vi "Update_FFID_Bkgnd_info.vi"(1 "First Bknd since calib":bool, 2 "c^2 (ppm^2)":dbl[](array[numeric]), 3 "Specific Bkgnd Meas?":bool, 4 "C (ppm)":dbl[](array[numeric])) -> ()   [LabVIEW 2021]
uses:
  Globals/Meas_global.vi
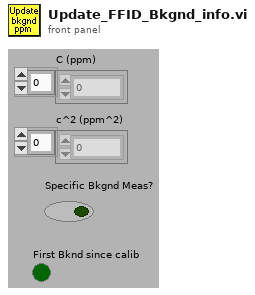
[diagram p1: front panel]
types:
  T1 = typedef "Analysis_info_cluster.ctl" = cluster{"Colour":u32, "Inst type":T2, "Inst name":string, "Symbol":string, "Code name":string, "Extra Info":string, "Inst Array":T3, "Extra Titles":string[], "Extra Values":string[], "U":dbl, "u^2":dbl, "u^3":dbl, "u^4":dbl, "Skew_u":dbl, "Kurt_u":dbl, "Sd Error in Mean":dbl, "% u'/U":dbl, "X":dbl, "Y":dbl, "Z":dbl, "Timescale integral Estimate":dbl, "Sd Error in Variance":dbl, "Calib File":path, "Calib Constants":dbl[], "Output Position":bool, "Stats":enum16{"None", "Basic", "Full"}, "Av Sampling Rate":dbl, "Av No of Samples":dbl, "Total Meas Time (s)":dbl, "ADAM Ch Name":string, "Max value":dbl, "Min value":dbl, "Req Sample Rate Hz":dbl, "Sync Delay Time (s)":dbl, "Ch No":i16, "Device":string, "Use Latest Calib":bool, "Port":string, "Metadata Ch Names":string[], "Metadata Ch Values":string[], "Label":string}
  T2 = typedef "Inst_type.ctl" = enum16{"Raw voltage", "Raw with zero offsetting", "Propeller anemometer", "Pressure Transducer", "Pitot-static tube", "Hot wire", "Cross wire 1", "Cross wire 2", "Generic Linear", "Generic Polynomial", "Generic BackPoly", "Fast FID", "Thermocouple", "Cold wire", "Pulsed Wire", "LDA Vel", "LDA Tran time", "LDA Arr time", "Microphone"}
  T3 = typedef "Instrument_Array.ctl" = enum16{"PWA", "LDA", "Analogue"}
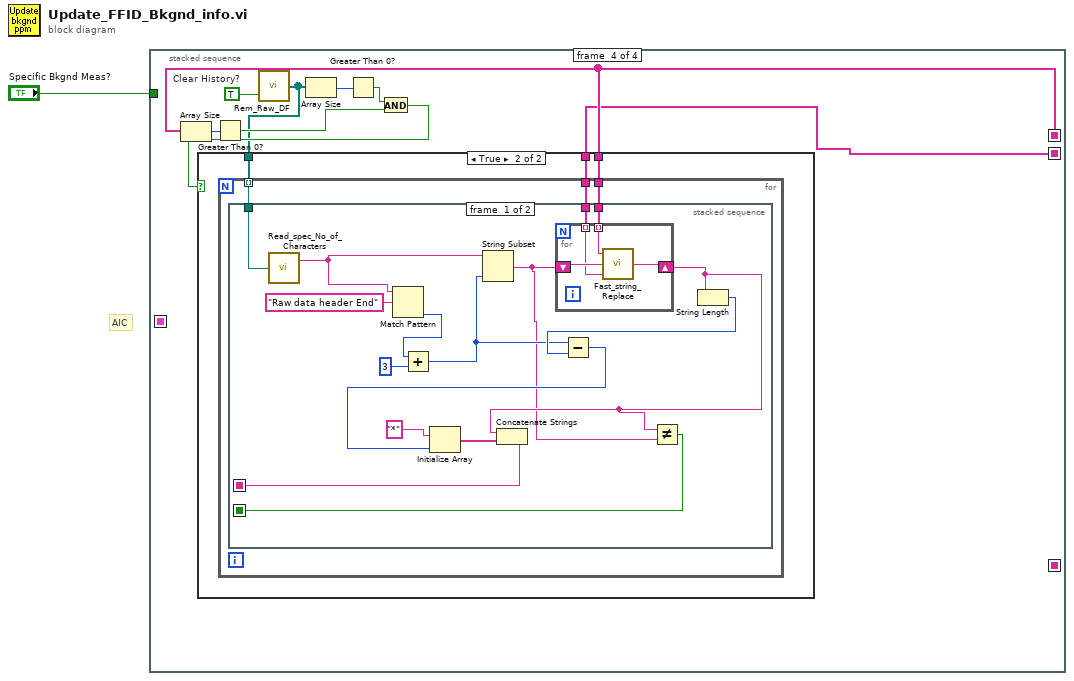
[diagram p0: block diagram]
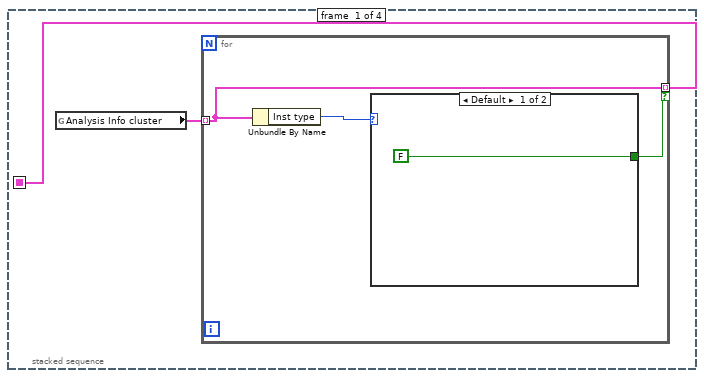
[diagram p2: hidden frame]
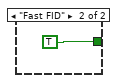
[diagram p3: hidden frame]
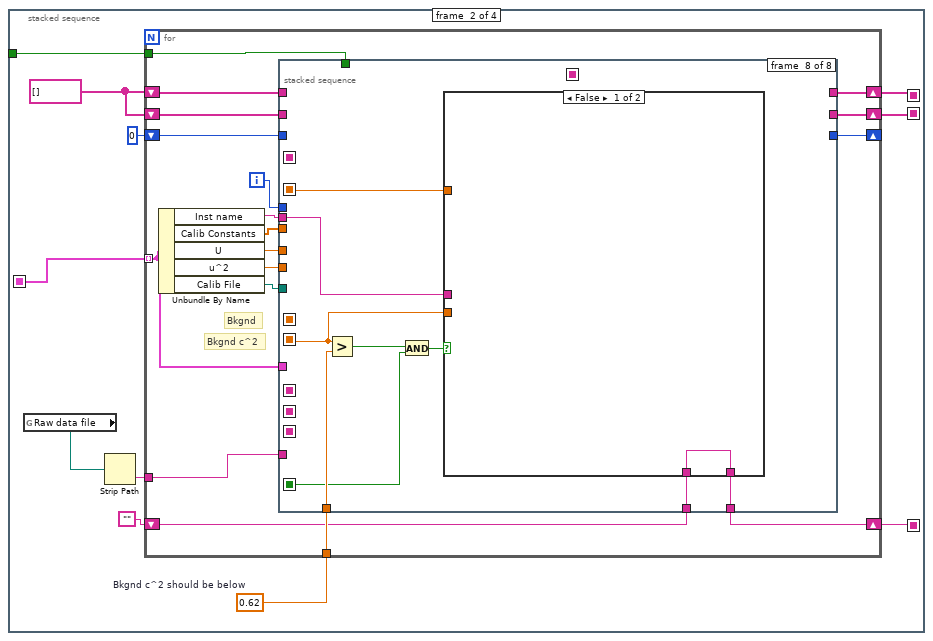
[diagram p4: hidden frame]
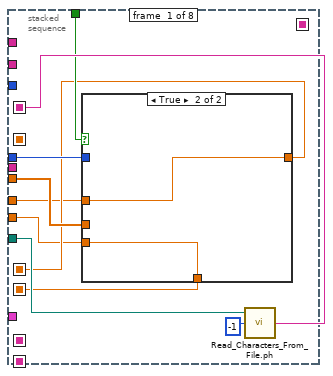
[diagram p5: hidden frame]
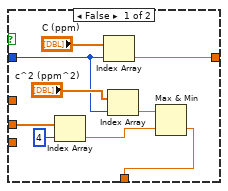
[diagram p6: hidden frame]
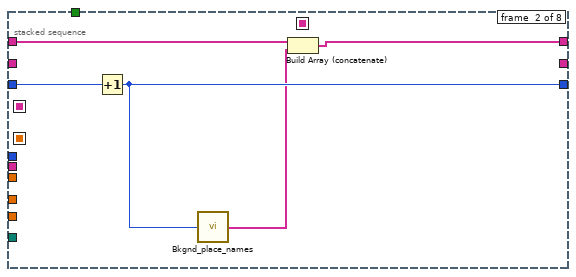
[diagram p7: hidden frame]
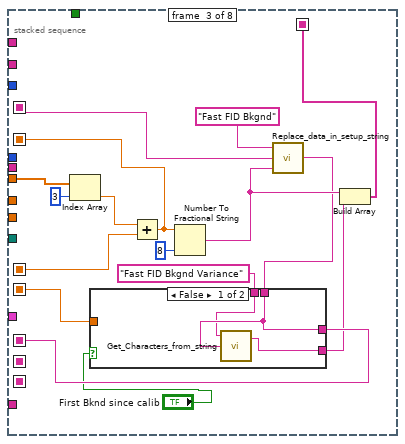
[diagram p8: hidden frame]
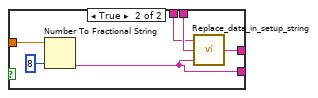
[diagram p9: hidden frame]
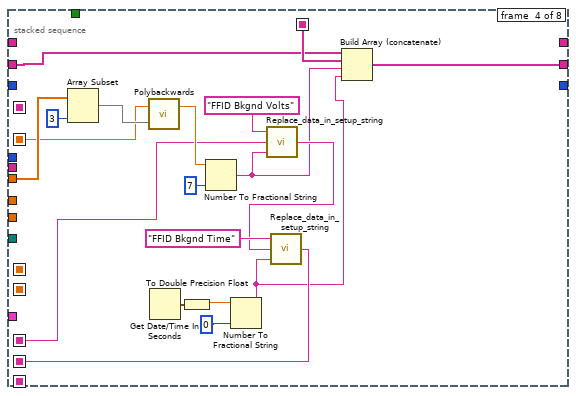
[diagram p10: hidden frame]
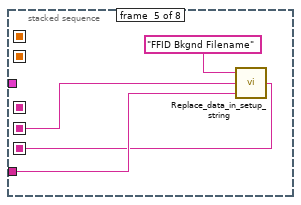
[diagram p11: hidden frame]
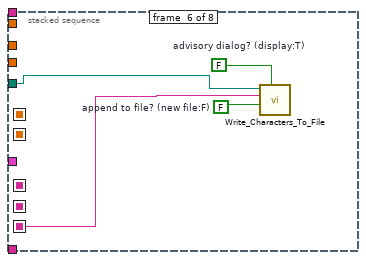
[diagram p12: hidden frame]
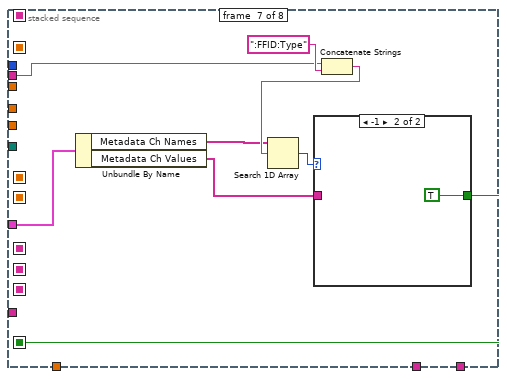
[diagram p13: hidden frame]
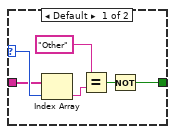
[diagram p14: hidden frame]
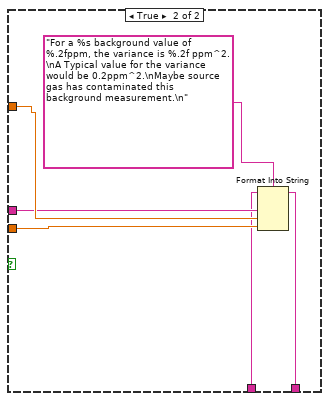
[diagram p15: hidden frame]
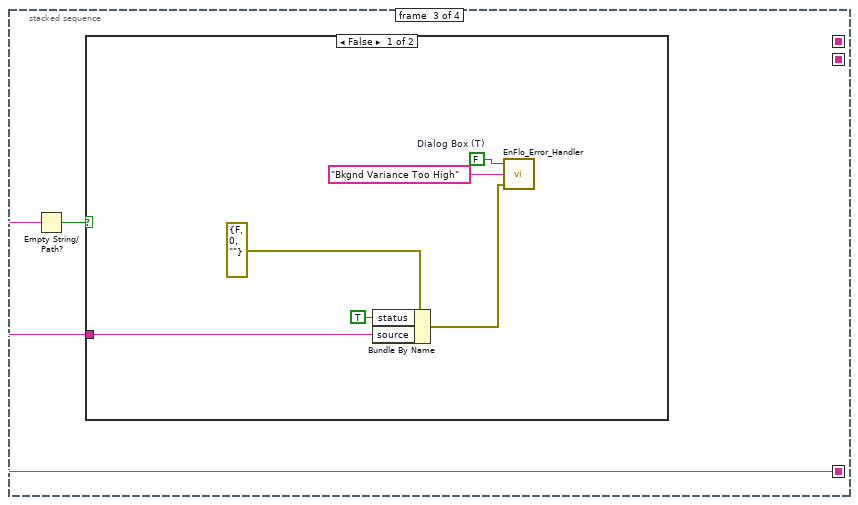
[diagram p16: hidden frame]
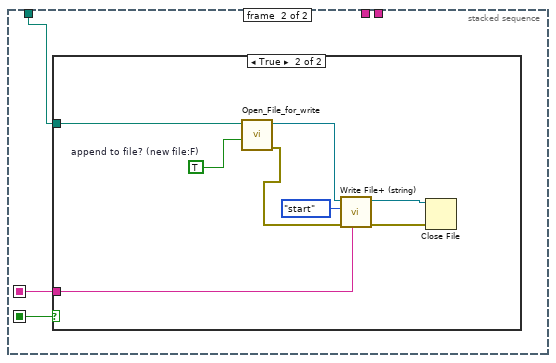
[diagram p19: hidden frame]
diagram:
  # "AIC"
  n1 = stacked-sequence {
    seq-local: [_ w15 _ _] -> [_ _ _ w157]
    seq-local: [_ w14 _ _] -> [_ _ _ w156]
    seq-local: [w2 _ _ _] -> [_ w12 _ _]
    seq-local: [_ w9 _ _] -> [_ _ w147 _]
    tunnel: "Specific Bkgnd Meas?" -> [_ w11 _ _]
    frame #0 {
      n2 = global read "Meas_global.vi" "Analysis Info cluster"() -> (w3:T1[])
      n3 = for {
        tunnel: w3 -> [w6] mode=indexing
        tunnel: [w6] -> w2 mode=indexing if=w4
        n4 = Unbundle By Name(w6) -> ("Inst type"=w5:T2)
        n5 = case shown="Default" w5 {
          tunnel: [FALSE TRUE] -> w4
          frame Default {
          }
          frame "Fast FID" {
          }
        }
      }
    }
    frame #1 {
      w13 = 0.62  # Bkgnd c^2 should be below
      w16 = string[] []
      n6 = global read "Meas_global.vi" "Raw data file"() -> (w19:path)
      n7 = Strip Path(path=w19) -> (name=w18:string)  [unwired: 1 out]
      n8 = for {
        tunnel: w18 -> [w37]
        shift-right: [w35] -> _
        shift-left: 0 -> [w36]
        shift-right: [w31] -> w14
        shift-left: w16 -> [w32]
        shift-right: [w33] -> w15
        shift-left: w16 -> [w34]
        tunnel: w13 -> [w30]
        tunnel: w12 -> [w22] mode=indexing
        tunnel: w11 -> [w29]
        shift-right: [w20] -> w9
        shift-left: "" -> [w21]
        i -> [w28]
        # "Bkgnd c^2"
        # "Bkgnd"
        n9 = Unbundle By Name(w22) -> ("Inst name"=w23:string, "Calib Constants"=w27:dbl[], "U"=w26:dbl, "u^2"=w24:dbl, "Calib File"=w25:path)
        n10 = stacked-sequence {
          seq-local: [w46 _ _ _ _ _ _ _] -> [_ _ w74 _ _ _ _ _]
          seq-local: [_ _ w73 _ _ _ _ _] -> [_ _ _ w96 _ _ _ _]
          seq-local: [_ _ w72 _ _ _ _ _] -> [_ _ _ w104 _ _ _ w139]
          seq-local: [_ _ _ w94 _ _ _ _] -> [_ _ _ _ w108 _ _ _]
          seq-local: [_ _ _ _ w109 _ _ _] -> [_ _ _ _ _ w113 _ _]
          seq-local: [_ _ w68 _ _ _ _ _] -> [_ _ _ w93 _ _ _ _]
          seq-local: [w43 _ _ _ _ _ _ _] -> [_ _ w67 _ _ _ _ w138]
          seq-local: [w40 _ _ _ _ _ _ _] -> [_ _ w66 _ _ _ _ _]
          seq-local: [_ _ _ _ _ _ w116 _] -> [_ _ _ _ _ _ _ w134]
          tunnel: w27 -> [w42 _ w79 w107 _ _ _ _]
          tunnel: w25 -> [w45 _ _ _ _ w112 _ _]
          tunnel: w37 -> [_ _ _ _ w110 _ _ _]
          tunnel: w36 -> [_ w63 _ _ _ _ _ _]
          tunnel: [_ w62 _ _ _ _ _ _] -> w35
          tunnel: w34 -> [_ w60 _ _ _ _ _ _]
          tunnel: [_ w59 _ _ _ _ _ _] -> w33
          tunnel: w32 -> [_ _ _ w90 _ _ _ _]
          tunnel: [_ _ _ w89 _ _ _ _] -> w31
          tunnel: w30 -> [_ _ _ _ _ _ _ w137]
          tunnel: w29 -> [w44 _ _ _ _ _ _ _]
          tunnel: w28 -> [w41 _ _ _ _ _ _ _]
          tunnel: w26 -> [w39 _ _ _ _ _ _ _]
          tunnel: w24 -> [w38 _ _ _ _ _ _ _]
          tunnel: w23 -> [_ _ _ _ _ _ w117 w136]
          tunnel: w22 -> [_ _ _ _ _ _ w120 _]
          tunnel: w21 -> [_ _ _ _ _ _ _ w132]
          tunnel: [_ _ _ _ _ _ _ w131] -> w20
          frame #0 {
            n11 = case shown="True" w44 {
              tunnel: [w48 w57] -> w43
              tunnel: w42 -> [w56 _]
              tunnel: w41 -> [w51 _]
              tunnel: [w53 w58] -> w40
              tunnel: w39 -> [_ w58]
              tunnel: w38 -> [_ w57]
              frame False {
                n12 = Index Array(array=w56, index=4) -> (element=w49:dbl)
                n13 = Index Array(array="C (ppm)", index=w51) -> (element=w53:dbl)
                n14 = Index Array(array="c^2 (ppm^2)", index=w51) -> (element=w50:dbl)
                n15 = Max & Min(x=w50, y=w49) -> (min(x,y)=w48:dbl)  [unwired: 1 out]
              }
              frame True {
              }
            }
            n16 = call "Read_Characters_From_File.ph.vi"("file path (dialog if empty)"=w45, "number of characters (all:-1)"=-1) -> ("character string"=w46:string)  [unwired: 7 out]
          }
          frame #1 {
            n17 = Increment(x=w63) -> (x+1=w62:i32)
            n18 = call "Bkgnd_place_names.vi"("Numeric"=w62) -> ("Array"=w61:string[])
            n19 = Build Array (concatenate)(w60, w61) -> (w59:string[])
          }
          frame #2 {
            n20 = Index Array(array=w79, index=3 ("Index")) -> (element=w77:dbl)
            n21 = Add(x=w77, y=w66) -> (x+y=w72:dbl)
            n22 = Number To Fractional String(number=w72, precision (6)=i16 8) -> (F-format string=w71:string)  [unwired: 2 out]
            n23 = call "Replace_data_in_setup_string.vi"("New data string"=w71, "Input string"=w74, "Variable name"="Fast FID Bkgnd") -> ("Appended string"=w70:string)
            n24 = case shown="False" "First Bknd since calib" {
              tunnel: [w82 w88] -> w73
              tunnel: w70 -> [w82 w86]
              tunnel: [w80 w85] -> w69
              tunnel: w67 -> [_ w84]
              tunnel: "Fast FID Bkgnd Variance" -> [w81 w83]
              frame False {
                n25 = call "Get_Characters_from_string.vi"("Input string"=w82, "Variable name"=w81) -> ("Value"=w80:string)  [unwired: 1 in, 1 out]
              }
              frame True {
                n26 = Number To Fractional String(number=w84, precision (6)=i16 8) -> (F-format string=w85:string)  [unwired: 2 out]
                n27 = call "Replace_data_in_setup_string.vi"("New data string"=w85, "Input string"=w86, "Variable name"=w83) -> ("Appended string"=w88:string)
              }
            }
            n28 = Build Array(w71, w69) -> (w68:string[])
          }
          frame #3 {
            n29 = Array Subset(array=w107, length=3 ("index")) -> (w105:dbl[])  [unwired: 1 in]
            n30 = call "Polybackwards.vi"("Coefficients"=w105, "Y input"=w104) -> ("X output"=w103:dbl)  [unwired: 1 out]
            n31 = Get Date/Time In Seconds() -> (seconds since 1Jan1904=w100:timestamp)
            n32 = To Double Precision Float(number=w100) -> (double precision float=w98:dbl)
            n33 = Number To Fractional String(number=w103, precision (6)=i16 7) -> (F-format string=w92:string)  [unwired: 2 out]
            n34 = Number To Fractional String(number=w98, precision (6)=i16 0) -> (F-format string=w91:string)  [unwired: 2 out]
            n35 = call "Replace_data_in_setup_string.vi"("New data string"=w92, "Input string"=w96, "Variable name"="FFID Bkgnd Volts") -> ("Appended string"=w95:string)
            n36 = call "Replace_data_in_setup_string.vi"("New data string"=w91, "Input string"=w95, "Variable name"="FFID Bkgnd Time") -> ("Appended string"=w94:string)
            n37 = Build Array (concatenate)(w90, w93, w92, w91) -> (w89:string[])
          }
          frame #4 {
            n38 = call "Replace_data_in_setup_string.vi"("New data string"=w110, "Input string"=w108, "Variable name"="FFID Bkgnd Filename") -> ("Appended string"=w109:string)
          }
          frame #5 {
            w114 = FALSE  # advisory dialog? (display:T)
            w115 = FALSE  # append to file? (new file:F)
            n39 = call "Write_Characters_To_File.vi"("file path (dialog if empty)"=w112, "advisory dialog? (display:T)"=w114, "character string"=w113, "append to file? (new file:F)"=w115) -> ()  [unwired: 1 in, 4 out]
          }
          frame #6 {
            n40 = Unbundle By Name(w120) -> ("Metadata Ch Names"=w119:string[], "Metadata Ch Values"=w118:string[])
            n41 = Concatenate Strings(w117, ":FFID:Type" ("string")) -> (w122:string)
            n42 = Search 1D Array(1D array=w119, element=w122) -> (index of element=w121:i32)  [unwired: 1 in]
            n43 = case shown="-1" w121 {
              selector: w121 -> [w129 _]
              tunnel: [w124 TRUE] -> w116
              tunnel: w118 -> [w128 _]
              frame Default {
                n44 = Index Array(array=w128, index=w129) -> (element=w127:string)
                n45 = Equal?(x="Other", y=w127) -> (x = y?=w125:bool)
                n46 = Not(x=w125) -> (.not. x?=w124:bool)
              }
              frame -1 {
              }
            }
          }
          frame #7 {
            n47 = Greater?(x=w138, y=w137) -> (0:w135:bool)
            n48 = And(x=w135, y=w134) -> (x .and. y?=w133:bool)
            n49 = case shown="False" w133 {
              tunnel: w138 -> [_ w146]
              tunnel: w139 -> [_ w145]
              tunnel: w136 -> [_ w143]
              tunnel: w132 -> [w140 w142]
              tunnel: [w140 w141] -> w131
              frame False {
              }
              frame True {
                n50 = Format Into String(format string="For a %s background value of %.2fppm, the variance is %.2f ppm^2.\nA Typical value for the variance would be 0.2ppm^2.\nMaybe source gas has contaminated this background measurement.\n", initial string=w142, w143, w145, w146) -> (resulting string=w141:string)  [unwired: 1 in, 1 out]
              }
            }
          }
        }
      }
    }
    frame #2 {
      n51 = Empty String/Path?(string/path=w147) -> (empty?=w148:bool)
      n52 = case shown="False" w148 {
        tunnel: w147 -> [w150 _]
        frame False {
          w153 = FALSE  # Dialog Box (T)
          n53 = Bundle By Name(cluster=errorcluster {"status"=FALSE, "code"=0, "source"=""} ("error in (no error)"), "status"=TRUE, "source"=w150) -> (w149:errorcluster)
          n54 = call "EnFlo_Error_Handler.vi"("error in (no error)"=w149, "Error Type"="Bkgnd Variance Too High", "Dialog Box (F)"=w153) -> ()  [unwired: 3 out]
        }
        frame True {
        }
      }
    }
    frame #3 {
      w155 = TRUE  # Clear History?
      n55 = Array Size(array=w157) -> (size(s)=w162:i32)
      n56 = Greater Than 0?(x=w162) -> (x > 0?=w160:bool)
      n57 = call "Rem_Raw_DF.vi"("Clear History?"=w155) -> ("List of Filenames"=w158:path[])  [unwired: 1 in]
      n58 = Array Size(array=w158) -> (size(s)=w163:i32)
      n59 = Greater Than 0?(x=w163) -> (x > 0?=w161:bool)
      n60 = And(x=w161, y=w160) -> (x .and. y?=w159:bool)
      n61 = case shown="True" w159 {
        tunnel: w158 -> [_ w166]
        tunnel: w157 -> [_ w165]
        tunnel: w156 -> [_ w164]
        frame False {
        }
        frame True {
          n62 = for {
            tunnel: w166 -> [w167] mode=indexing
            tunnel: w165 -> [w169]
            tunnel: w164 -> [w168]
            n63 = stacked-sequence {
              seq-local: [w173 _] -> [_ w191]
              seq-local: [w171 _] -> [_ w190]
              tunnel: w169 -> [w181 _]
              tunnel: w168 -> [w180 _]
              tunnel: w167 -> [w174 w192]
              frame #0 {
                n64 = call "Read_spec_No_of_Characters.vi"("Filename"=w174) -> ("character string"=w182:string)  [unwired: 1 out]
                n65 = Match Pattern(string=w182, regular expression="Raw data header End") -> (offset past match=w184:i32)  [unwired: 4 out]
                n66 = Add(x=w184, y=3) -> (x+y=w178:i32)
                n67 = String Subset(string=w182, length (rest)=w178) -> (substring=w170:string)  [unwired: 1 out]
                n68 = for {
                  shift-right: [w188] -> w172
                  shift-left: w170 -> [w189]
                  tunnel: w181 -> [w187] mode=indexing
                  tunnel: w180 -> [w186] mode=indexing
                  n69 = call "Fast_string_Replace.vi"("Replace match with:"=w186, "Input String"=w189, "regular expression"=w187) -> ("Output String"=w188:string)  [unwired: 2 out]
                }
                n70 = Not Equal?(x=w172, y=w170) -> (x != y?=w171:bool)
                n71 = String Length(string=w172) -> (length=w179:i32)
                n72 = Subtract(x=w178, y=w179) -> (x-y=w176:i32)
                n73 = Initialize Array("*", w176) -> (w175:string[])
                n74 = Concatenate Strings(w172, w175) -> (w173:string)
              }
              frame #1 {
                n75 = case shown="True" w190 {
                  tunnel: w192 -> [_ w200]
                  tunnel: w191 -> [_ w193]
                  frame False {
                  }
                  frame True {
                    w199 = TRUE  # append to file? (new file:F)
                    n76 = call "Open_File_for_write.vi"("append to file? (new file:F)"=w199, "file path"=w200) -> ("error out"=w196:errorcluster, "refnum"=w197:refnum<file>)  [unwired: 1 in, 7 out]
                    n77 = call <vilib>:"Write File+ (string).vi"("string"=w193, "error in (no error)"=w196, "pos mode (rel. to end:1)"=enum16{"start", "end", "current"}."start", "refnum"=w197) -> ("error out"=w194:errorcluster, "dup refnum"=w195:refnum<file>)  [unwired: 1 in, 3 out]
                    n78 = Close File(refnum=w195, error in=w194) -> ()  [unwired: 2 out]
                  }
                }
              }
            }
          }
        }
      }
    }
  }
